vi "Calculate Graph Position Indicators.vi"(8 "Pattern offset":dbl, 9 "Pattern teeth":u16, 10 "Pattern length":dbl, 11 "Cursor position":dbl) -> (2 "Tooth":u16, 3 "Offset":dbl format="%#_6f")   [LabVIEW 2020, in "Engine Simulation Toolkit System Explorer.lvlib"]
uses:
  Engine Simulation Toolkit System Explorer.lvlib
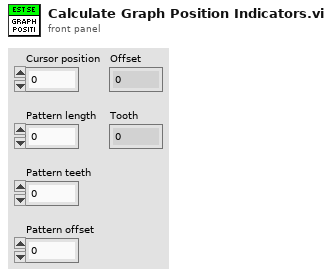
[diagram p1: front panel]
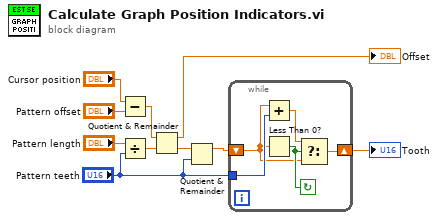
[diagram p0: block diagram]
diagram:
  n1 = Subtract(x="Cursor position", y="Pattern offset") -> (x-y=w1:dbl)
  n2 = Divide(x="Pattern length", y="Pattern teeth") -> (x/y=w2:dbl)
  n3 = Quotient & Remainder(x=w1, y=w2) -> (x-y*floor(x/y)=→"Offset":dbl, floor(x/y)=w3:dbl)
  n4 = Quotient & Remainder(x=w3, y="Pattern teeth") -> (x-y*floor(x/y)=w4:dbl)  [unwired: 1 out]
  n5 = while {
    tunnel: "Pattern teeth" -> [w12]
    shift-right: [w14] -> w9
    shift-left: w4 -> [w11]
    stop <- w15 continue-if-true
    n6 = Add(x=w11, y=w12) -> (x+y=w13:dbl)
    n7 = Less Than 0?(x=w11) -> (x < 0?=w15:bool)
    n8 = Select(t=w13, s=w15, f=w11) -> (s? t:f=w14:dbl)
  }
  "Tooth" <- w9
